vi "Puff_Dose.vi"() -> (5 "Plug in titles":string[](array[string]), 7 "Plug in values":string[](array[string]))   [LabVIEW 2014]
uses:
  Controls/Post_Process.ctl
  <vilib>/Analysis/baseanly.llb/Mean (DBL).vi
  Globals/Meas_global.vi
  Globals/Plug_in_data_global.vi
  <vilib>/Analysis/NI_AALBase.lvlib
panel:
  out "Active Trace length":i32
  out "Background time used (s)":dbl
  out "Delta T":dbl
  out "Min Dose":dbl
  out "Stats Names":string[](array[string])
  out "Stats values":string[](array[string])
  in  "File Extension":string=".xls"
  in  "Save Puff file":bool
  out "Bkgnd value (ppm)":dbl format="%0.2f"
  out "Array":dbl[][](array[numeric])
  out "Puff Number":i32=51
  out "XY Graph":cluster{"Time (s)":dbl[], "Eng Values":dbl[]}[](graph)
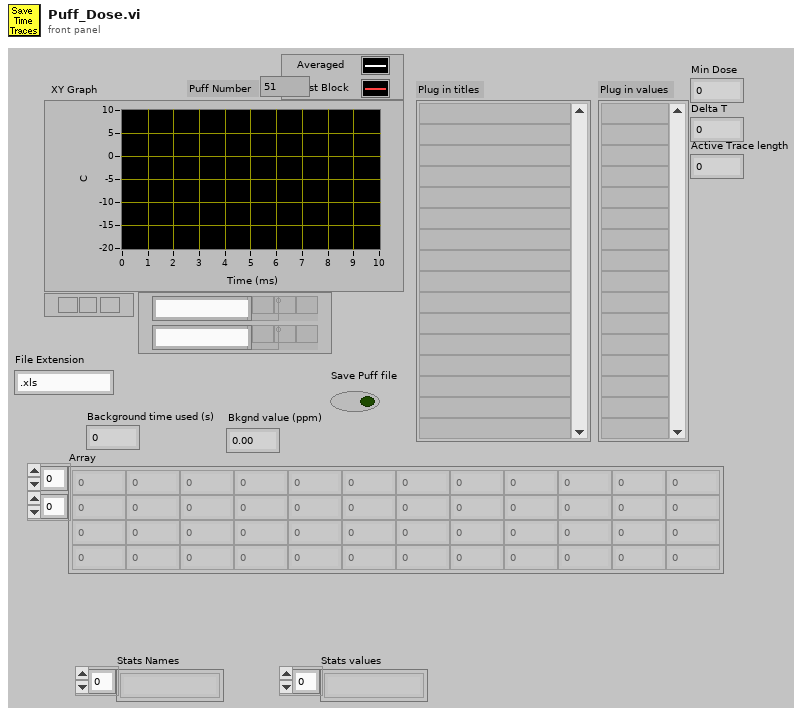
[diagram p1: front panel]
types:
  T1 = typedef "Analysis_info_cluster.ctl" = cluster{"Colour":u32, "Inst type":T2, "Inst name":string, "Symbol":string, "Code name":string, "Extra Info":string, "Inst Array":T3, "Extra Titles":string[], "Extra Values":string[], "U":dbl, "u^2":dbl, "u^3":dbl, "u^4":dbl, "Skew_u":dbl, "Kurt_u":dbl, "Sd Error in Mean":dbl, "% u'/U":dbl, "X":dbl, "Y":dbl, "Z":dbl, "Timescale integral to 25%":dbl, "Sd Error in Variance":dbl, "Calib File":path, "Calib Constants":dbl[], "Output Position":bool, "Full Stats":bool, "Av Sampling Rate":dbl, "Av No of Samples":dbl, "Total Meas Time (s)":dbl, "ADAM Ch Name":string}
  T2 = typedef "Inst_type.ctl" = enum16{"Propeller anemometer", "Raw voltage", "Pressure Transducer", "Pitot-static tube", "Preston tube", "Hot wire", "Cross wire 1", "Cross wire 2", "Generic Linear", "Generic Polynomial", "Generic BackPoly", "Fast FID", "Thermocouple", "Cold wire", "Pulsed Wire", "LDA Vel", "LDA Tran time", "LDA Arr time"}
  T3 = typedef "Instrument_Array.ctl" = enum16{"PWA", "LDA", "Analogue"}
  T4 = typedef "Post_Process.ctl" = enum16{"Take New Data", "Post Process Raw Data File"}
  T5 = enum16{"Save no data", "Save data in new files", "Save data in existing files"}
  T6 = typedef "Time_Trace_Cluster.ctl" = cluster{"Weighting":dbl[], "Time (s)":dbl[], "Voltage":dbl[], "Eng Values":dbl[]}
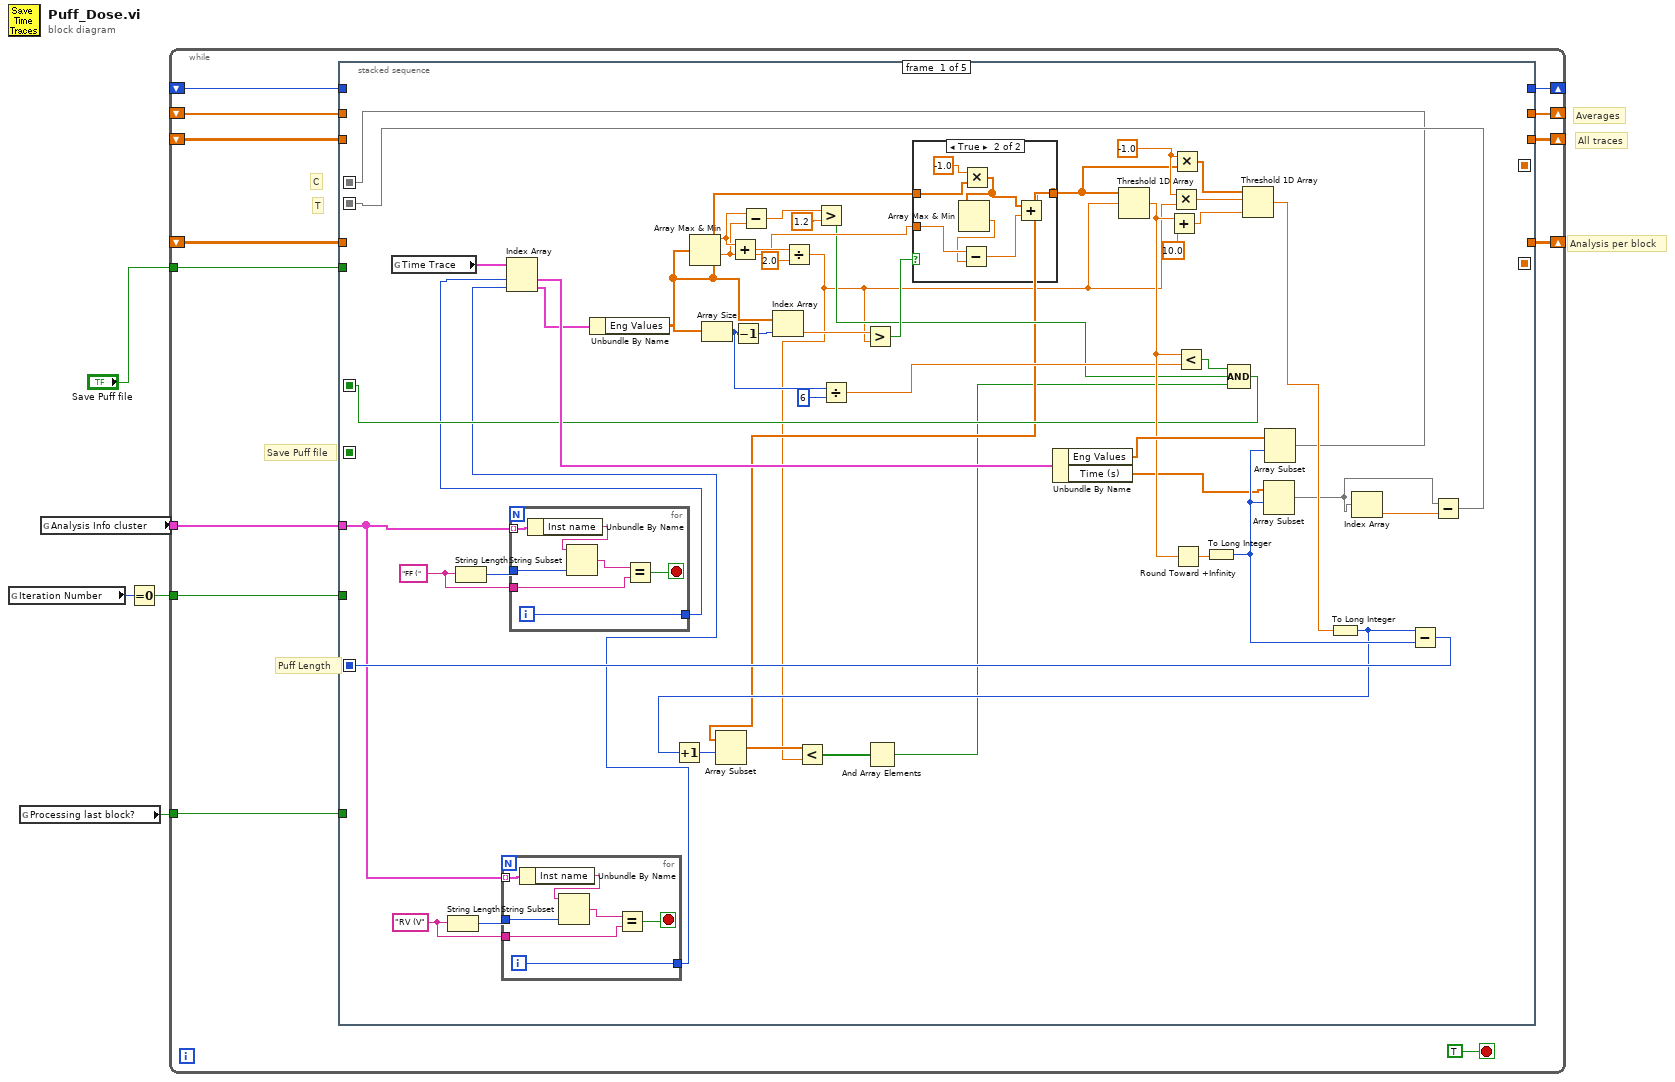
[diagram p0: block diagram]
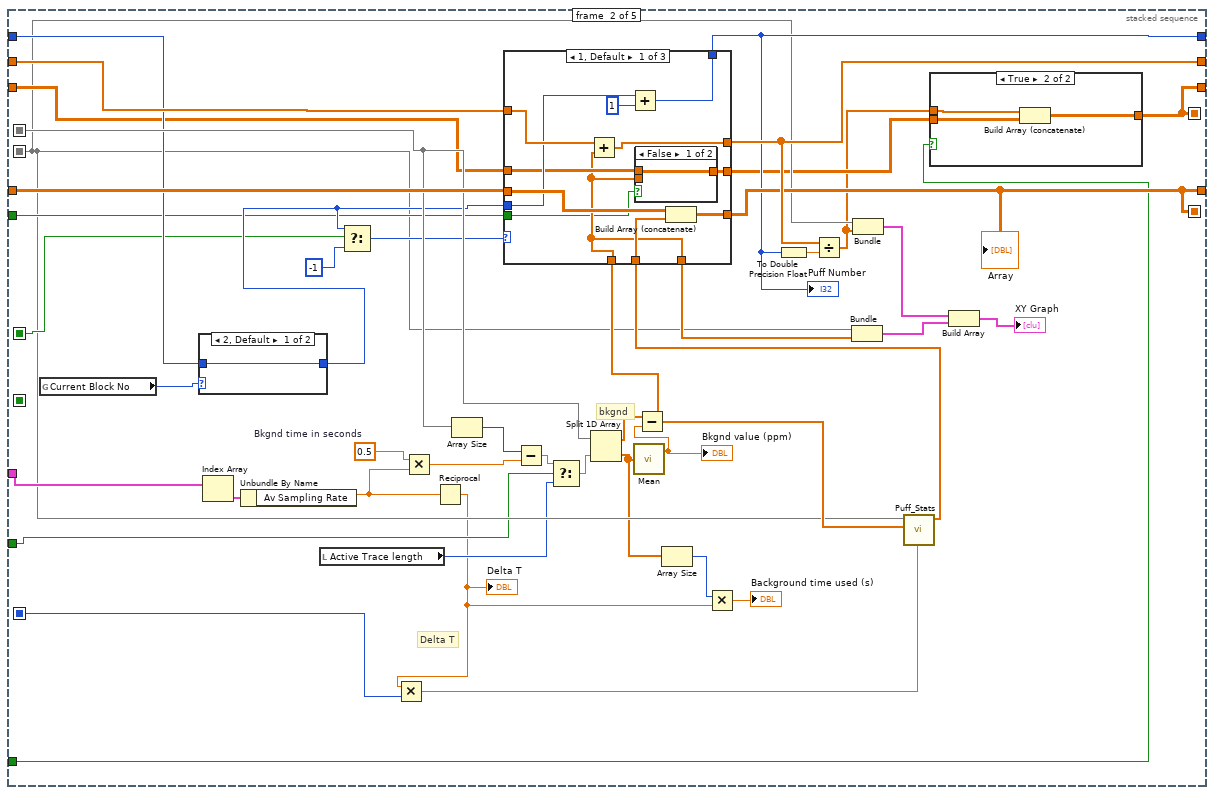
[diagram p3: hidden frame]
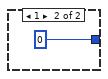
[diagram p5: hidden frame]
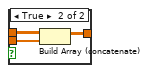
[diagram p6: hidden frame]
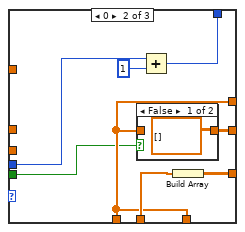
[diagram p7: hidden frame]
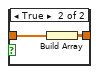
[diagram p8: hidden frame]
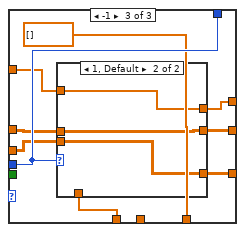
[diagram p9: hidden frame]
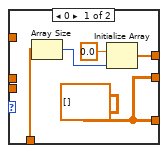
[diagram p10: hidden frame]
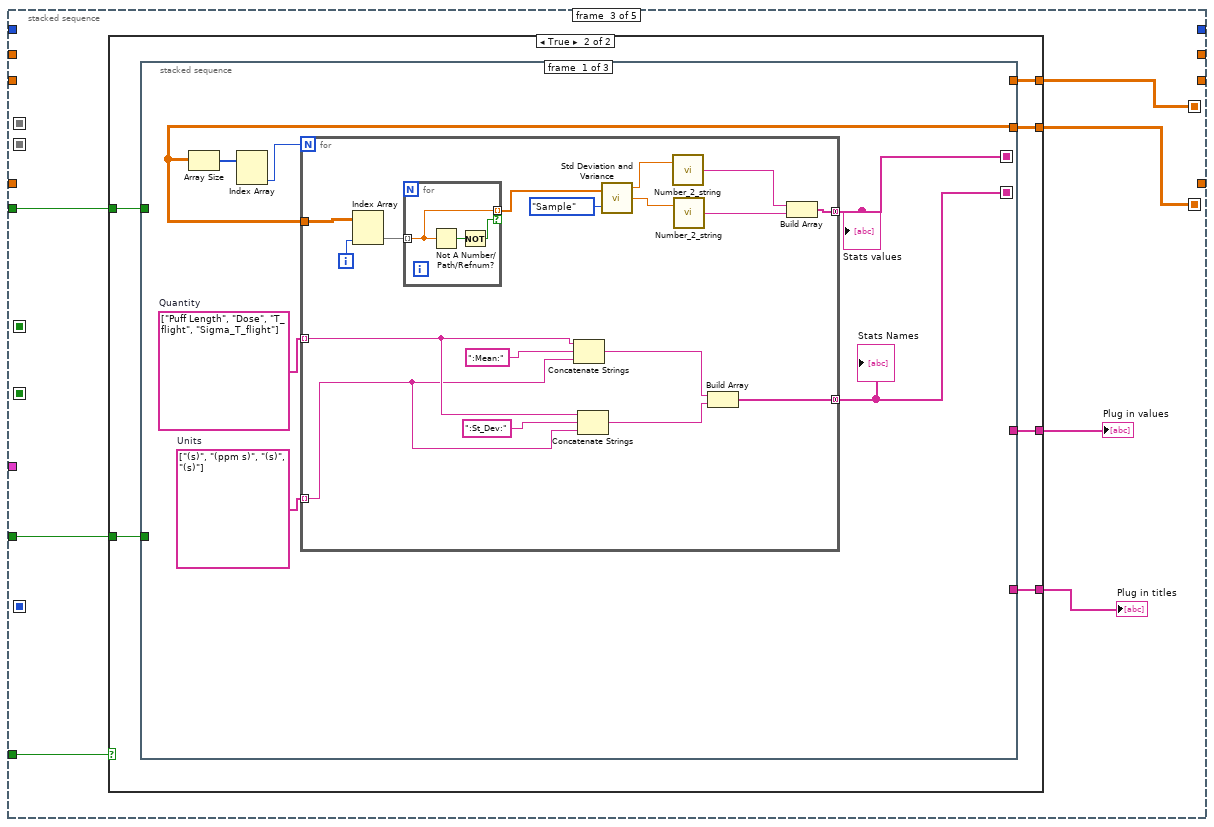
[diagram p11: hidden frame]
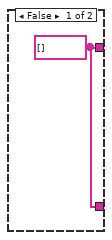
[diagram p12: hidden frame]
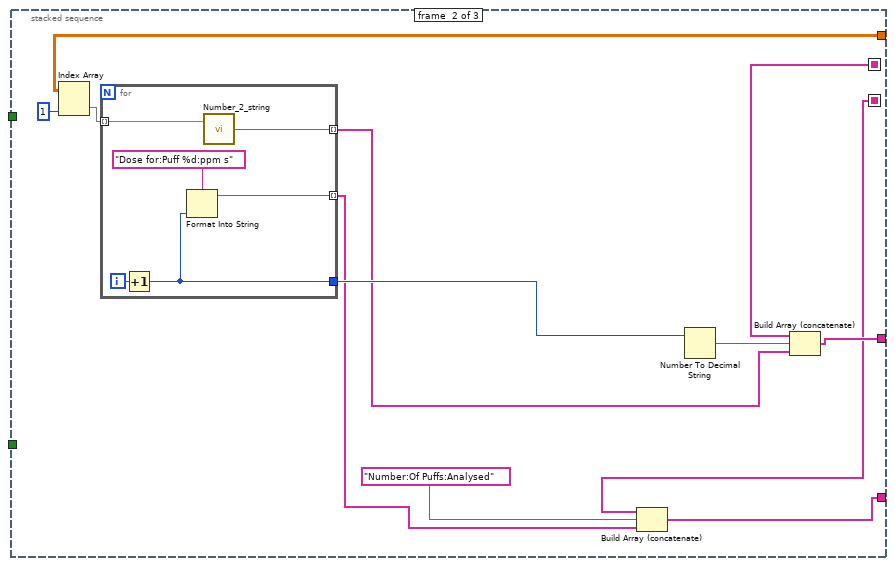
[diagram p13: hidden frame]
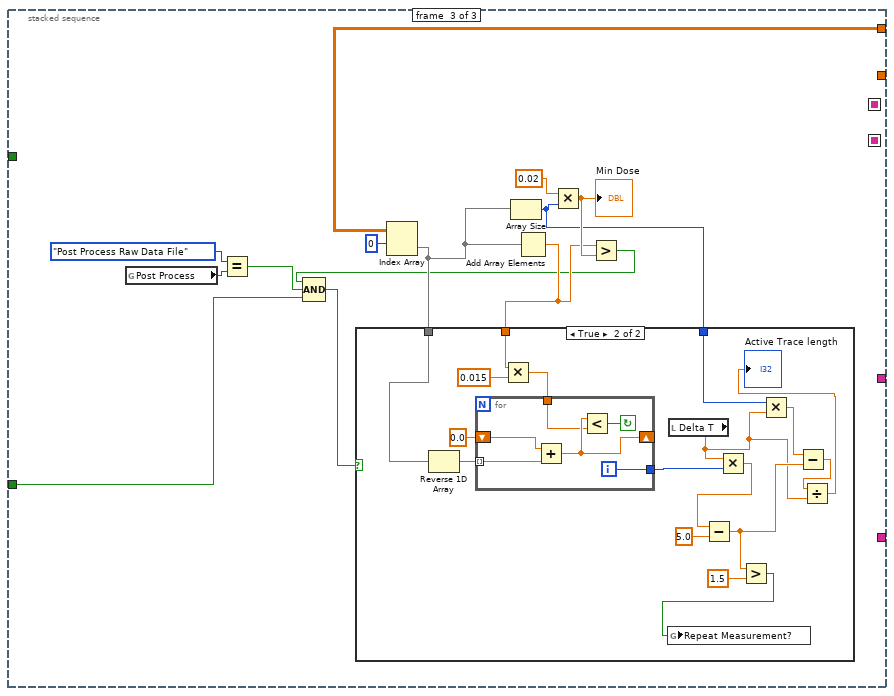
[diagram p14: hidden frame]
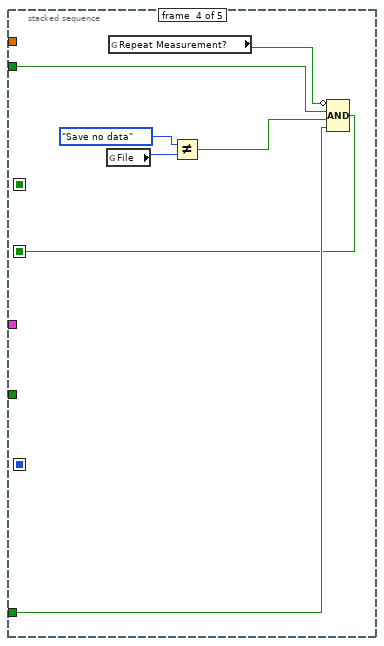
[diagram p16: hidden frame]
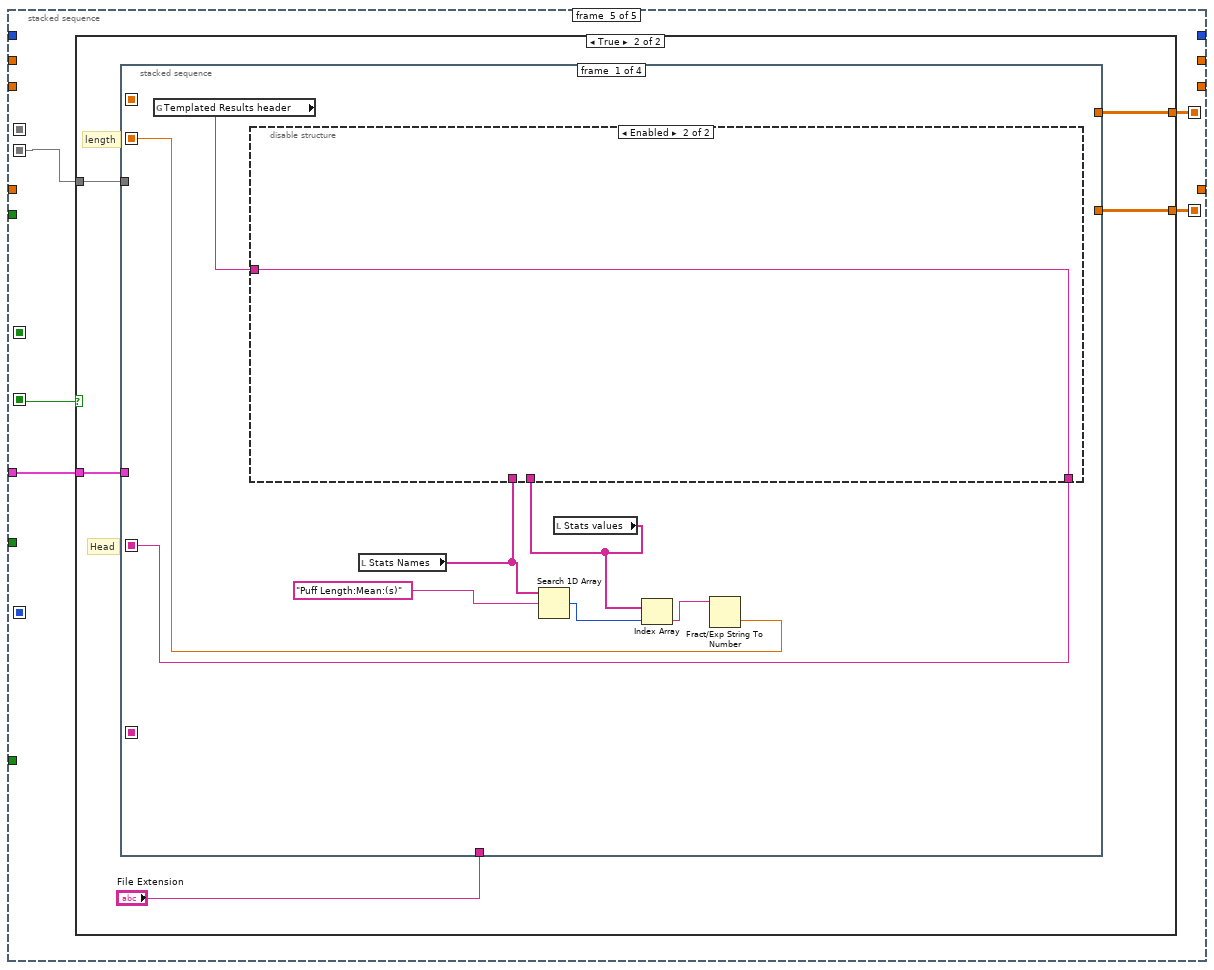
[diagram p17: hidden frame]
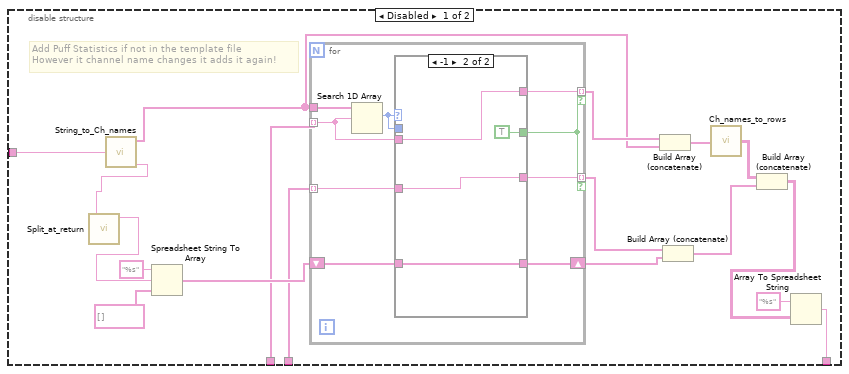
[diagram p19: hidden frame]
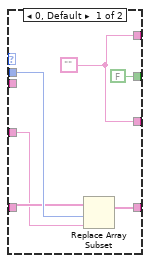
[diagram p20: hidden frame]
diagram:
  # "Averages"
  # "All traces"
  # "Analysis per block"
  n1 = global read "Meas_global.vi" "Iteration Number"() -> (w2:i32)
  n2 = global read "Meas_global.vi" "Processing last block?"() -> (w3:bool)
  n3 = global read "Meas_global.vi" "Analysis Info cluster"() -> (w5:T1[])
  n4 = Equal To 0?(x=w2) -> (x = 0?=w1:bool)
  n5 = while {
    shift-right: [w16] -> _
    shift-left: _ -> [w18]
    shift-right: [w14] -> _
    shift-left: _ -> [w15]
    tunnel: w5 -> [w13]
    shift-right: [w11] -> _
    shift-left: _ -> [w12]
    shift-right: [w10] -> _
    shift-left: _ -> [w9]
    tunnel: "Save Puff file" -> [w8]
    tunnel: w3 -> [w7]
    tunnel: w1 -> [w6]
    stop <- TRUE stop-if-true
    # "Save Puff file"
    # "Puff Length"
    # "T"
    # "C"
    n6 = stacked-sequence {
      seq-local: [_ w121 _ _ _] -> [_ _ w190 _ w289]
      seq-local: [w34 _ _ _ _] -> [_ w120 _ _ _]
      seq-local: [w35 _ _ _ _] -> [_ w103 _ _ w287]
      seq-local: [w33 _ _ _ _] -> [_ w118 _ _ _]
      seq-local: [w38 _ _ _ _] -> [_ w109 _ _ _]
      seq-local: [_ w99 _ _ _] -> [_ _ w184 _ w290]
      seq-local: [_ _ _ w280 _] -> [_ _ _ _ w286]
      tunnel: w18 -> [_ w117 _ _ _]
      tunnel: [_ w132 _ _ _] -> w16
      tunnel: w15 -> [_ w122 _ _ _]
      tunnel: [_ w121 _ _ _] -> w14
      tunnel: w13 -> [w21 w119 _ _ w288]
      tunnel: w12 -> [_ w115 _ _ _]
      tunnel: [_ w114 _ _ _] -> w11
      tunnel: [_ w99 _ _ _] -> w10
      tunnel: w9 -> [_ w105 _ _ _]
      tunnel: w8 -> [_ w104 w187 w283 _]
      tunnel: w7 -> [_ w102 w186 w281 _]
      tunnel: w6 -> [_ w96 w185 _ _]
      frame #0 {
        w23 = "RV (V"
        w58 = -1.0
        w65 = "FF ("
        n7 = global read "Meas_global.vi" "Time Trace"() -> (w67:T6[])
        n8 = String Length(string=w23) -> (length=w22:i32)
        n9 = String Length(string=w65) -> (length=w66:i32)
        n10 = for {
          tunnel: w21 -> [w74] mode=indexing
          tunnel: w22 -> [w73]
          tunnel: w23 -> [w70]
          tunnel: [w68] -> w20
          i -> [w68]
          stop <- w69 stop-if-true
          n11 = Unbundle By Name(w74) -> ("Inst name"=w72:string)
          n12 = String Subset(string=w72, length (rest)=w73) -> (substring=w71:string)  [unwired: 1 in]
          n13 = Equal?(x=w71, y=w70) -> (x = y?=w69:bool)
        }
        n14 = for {
          tunnel: w21 -> [w89] mode=indexing
          tunnel: w66 -> [w88]
          tunnel: w65 -> [w85]
          tunnel: [w83] -> w19
          i -> [w83]
          stop <- w84 stop-if-true
          n15 = Unbundle By Name(w89) -> ("Inst name"=w87:string)
          n16 = String Subset(string=w87, length (rest)=w88) -> (substring=w86:string)  [unwired: 1 in]
          n17 = Equal?(x=w86, y=w85) -> (x = y?=w84:bool)
        }
        n18 = Index Array(array=w67, index #1=w19, index #2=w20) -> (element #1=w64:T6, element #2=w63:T6)
        n19 = Unbundle By Name(w63) -> ("Eng Values"=w30:dbl[])
        n20 = Array Max & Min(array=w30) -> (max value=w48:dbl, min value=w47:dbl)  [unwired: 2 out]
        n21 = Array Size(array=w30) -> (size(s)=w43:i32)
        n22 = Add(x=w48, y=w47) -> (x+y=w62:dbl)
        n23 = Decrement(x=w43) -> (x-1=w52:i32)
        n24 = Subtract(x=w48, y=w47) -> (x-y=w46:dbl)
        n25 = Index Array(array=w30, index=w52) -> (element=w51:dbl)
        n26 = Divide(x=w62, y=2.0) -> (x/y=w26:dbl)
        n27 = Greater?(x=w46, y=1.2) -> (0:w39:bool)
        n28 = Divide(x=w43, y=6) -> (x/y=w41:dbl)
        n29 = Greater?(x=w51, y=w26) -> (0:w50:bool)
        n30 = case shown="True" w50 {
          tunnel: w30 -> [w75 w81]
          tunnel: [w75 w76] -> w28
          tunnel: w47 -> [_ w80]
          frame False {
          }
          frame True {
            n31 = Multiply(x=-1.0, y=w81) -> (x*y=w77:dbl[])
            n32 = Array Max & Min(array=w77) -> (min value=w79:dbl)  [unwired: 3 out]
            n33 = Subtract(x=w80, y=w79) -> (x-y=w78:dbl)
            n34 = Add(x=w77, y=w78) -> (x+y=w76:dbl[])
          }
        }
        n35 = Unbundle By Name(w64) -> ("Eng Values"=w55:dbl[], "Time (s)"=w31:dbl[])
        n36 = Threshold 1D Array(2:w26, 3:w28) -> (0:w44:dbl)  [unwired: 1 in]
        n37 = Add(x=w44, y=10.0) -> (x+y=w60:dbl)
        n38 = Multiply(x=w58, y=w26) -> (x*y=w57:dbl)
        n39 = Multiply(x=w58, y=w28) -> (x*y=w49:dbl[])
        n40 = Round Toward +Infinity(x=w44) -> (ceil(x): smallest int >= x=w56:dbl)
        n41 = Less?(x=w44, y=w41) -> (x < y?=w40:bool)
        n42 = To Long Integer(number=w56) -> (32bit integer=w53:i32)
        n43 = Threshold 1D Array(1:w60, 2:w57, 3:w49) -> (0:w54:dbl)
        n44 = Array Subset(array=w31, index=w53) -> (w36:dbl[])  [unwired: 1 in]
        n45 = Array Subset(array=w55, index=w53) -> (w34:dbl[])  [unwired: 1 in]
        n46 = To Long Integer(number=w54) -> (32bit integer=w32:i32)
        n47 = Increment(x=w32) -> (x+1=w29:i32)
        n48 = Array Subset(array=w28, index=w29) -> (w27:dbl[])  [unwired: 1 in]
        n49 = Less?(x=w27, y=w26) -> (x < y?=w25:bool[])
        n50 = And Array Elements(Boolean array=w25) -> (logical AND=w24:bool)
        n51 = Compound Arithmetic op=AND(w40, w39, w24) -> (w38:bool)
        n52 = Index Array(array=w36) -> (element=w37:dbl)  [unwired: 1 in]
        n53 = Subtract(x=w32, y=w53) -> (x-y=w33:i32)
        n54 = Subtract(x=w36, y=w37) -> (x-y=w35:dbl[])
      }
      frame #1 {
        w90 = 0.5  # Bkgnd time in seconds
        # "bkgnd"
        # "Delta T"
        n55 = global read "Meas_global.vi" "Current Block No"() -> (w116:i32)
        n56 = case shown="2, Default" w116 {
          tunnel: [w138 0] -> w113
          tunnel: w115 -> [w138 _]
          frame 2, Default {
          }
          frame 1 {
          }
        }
        n57 = Index Array(array=w119) -> (element=w128:T1)  [unwired: 1 in]
        n58 = Unbundle By Name(w128) -> ("Av Sampling Rate"=w123:dbl)
        n59 = local read "Active Trace length"() -> (w95:i32)
        n60 = Select(t=w113, s=w109, f=-1) -> (s? t:f=w111:i32)
        n61 = Multiply(x=w90, y=w123) -> (x*y=w126:dbl)
        n62 = Reciprocal(x=w123) -> (1/x=w91:dbl)
        "Delta T" <- w91
        n63 = Multiply(x=w91, y=w118) -> (x*y=w108:dbl)
        n64 = Array Size(array=w120) -> (size(s)=w127:i32)
        n65 = Subtract(x=w127, y=w126) -> (x-y=w98:dbl)
        n66 = Select(t=w98, s=w96, f=w95) -> (s? t:f=w97:dbl)
        n67 = Split 1D Array(array=w120, index=w97) -> (first subarray=w124:dbl[], second subarray=w94:dbl[])
        n68 = call-poly <vilib>:"Mean.vi"("X"=w94) -> ("mean"=w125:dbl)  [unwired: 1 out]
        "Bkgnd value (ppm)" <- w125
        n69 = Subtract(x=w124, y=w125) -> (x-y=w107:dbl[])
        n70 = Array Size(array=w94) -> (size(s)=w93:i32)
        n71 = Multiply(x=w93, y=w91) -> (x*y=→"Background time used (s)":dbl)
        n72 = call "Puff_Stats.vi"("Puff release time (s)"=w108, "Concentrations"=w107, "Time (s)"=w103) -> ("Stats"=w110:dbl[])  [unwired: 8 in]
        n73 = case shown="1, Default" w111 {
          tunnel: [w150 w158 w174] -> w132
          tunnel: w117 -> [w151 _ w173]
          tunnel: w110 -> [w149 w163 _]
          tunnel: [w148 w162 w169] -> w121
          tunnel: w122 -> [w147 _ w172]
          tunnel: w113 -> [w144 w161 w175]
          tunnel: [w145 w159 w175] -> w114
          tunnel: w107 -> [w142 w158 w171]
          tunnel: [w142 w158 dbl[] []] -> w106
          tunnel: [w141 w157 w168] -> w101
          tunnel: w105 -> [w143 _ w167]
          tunnel: w104 -> [w140 w156 _]
          frame 1, Default {
            n74 = Add(x=w151, y=w142) -> (x+y=w150:dbl[])
            n75 = Add(x=w144, y=1) -> (x+y=w145:i32)
            n76 = case shown="False" w140 {
              tunnel: w143 -> [w152 w155]
              tunnel: w142 -> [_ w154]
              tunnel: [w152 w153] -> w141
              frame False {
              }
              frame True {
                n77 = Build Array (concatenate)(w155, w154) -> (w153:dbl[][])
              }
            }
            n78 = Build Array (concatenate)(w147, w149) -> (w148:dbl[][])
          }
          frame 0 {
            n79 = case shown="False" w156 {
              tunnel: w158 -> [_ w166]
              tunnel: [dbl[][] [] w165] -> w157
              frame False {
              }
              frame True {
                n80 = Build Array(w166) -> (w165:dbl[][])
              }
            }
            n81 = Add(x=w161, y=1) -> (x+y=w159:i32)
            n82 = Build Array(w163) -> (w162:dbl[][])
          }
          frame -1 {
            n83 = case shown="1, Default" w175 {
              tunnel: w171 -> [w180 _]
              tunnel: [w177 w183] -> w174
              tunnel: [w176 w182] -> w169
              tunnel: w173 -> [_ w183]
              tunnel: w172 -> [_ w182]
              tunnel: [w176 w181] -> w168
              tunnel: w167 -> [_ w181]
              frame 0 {
                w176 = dbl[][] []
                n84 = Array Size(array=w180) -> (size(s)=w179:i32)
                n85 = Initialize Array(0.0 ("element"), w179) -> (w177:dbl[])
              }
              frame 1, Default {
              }
            }
          }
        }
        "Puff Number" <- w114
        "Array" <- w121
        n86 = To Double Precision Float(number=w114) -> (double precision float=w133:dbl)
        n87 = Divide(x=w132, y=w133) -> (x/y=w100:dbl[])
        n88 = Bundle(w103, w106) -> (w131:cluster{dbl[], dbl[]})  [unwired: 1 in]
        n89 = Bundle(w103, w100) -> (w130:cluster{dbl[], dbl[]})  [unwired: 1 in]
        n90 = case shown="True" w102 {
          tunnel: w101 -> [w134 w137]
          tunnel: w100 -> [_ w136]
          tunnel: [w134 w135] -> w99
          frame False {
          }
          frame True {
            n91 = Build Array (concatenate)(w136, w137) -> (w135:dbl[][])
          }
        }
        n92 = Build Array(w130, w131) -> (→"XY Graph":cluster{dbl[], dbl[]}[])
      }
      frame #2 {
        n93 = case shown="True" w186 {
          tunnel: w190 -> [_ w197]
          tunnel: [w191 w196] -> w189
          tunnel: [w191 w195] -> w188
          tunnel: w187 -> [_ w194]
          tunnel: w185 -> [_ w193]
          tunnel: w184 -> [_ w192]
          frame False {
            w191 = string[] []
          }
          frame True {
            n94 = stacked-sequence {
              seq-local: [w199 _ _] -> [_ w231 _]
              seq-local: [w198 _ _] -> [_ w230 _]
              tunnel: w197 -> [w202 w234 _]
              tunnel: [_ w236 _] -> w196
              tunnel: [_ w235 _] -> w195
              tunnel: w194 -> [_ _ _]
              tunnel: w193 -> [_ _ w252]
              tunnel: w192 -> [_ _ w251]
              frame #0 {
                w200 = string[] ["(s)", "(ppm s)", "(s)", "(s)"]  # Units
                w201 = string[] ["Puff Length", "Dose", "T_flight", "Sigma_T_flight"]  # Quantity
                n95 = Array Size(array=w202) -> (size(s)=w204:i32[])
                n96 = Index Array(array=w204) -> (element #2=w203:i32)  [unwired: 2 in, 1 out]
                n97 = for {
                  N: w203 -> [_]
                  tunnel: w202 -> [w221]
                  tunnel: w201 -> [w212] mode=indexing
                  tunnel: w200 -> [w211] mode=indexing
                  tunnel: [w208] -> w199 mode=concatenating
                  tunnel: [w207] -> w198 mode=concatenating
                  i -> [w220]
                  n98 = Index Array(array=w221, index (col)=w220) -> (element=w206:dbl[])  [unwired: 1 in]
                  n99 = for {
                    tunnel: w206 -> [w224] mode=indexing
                    tunnel: [w224] -> w205 mode=indexing if=w222
                    n100 = Not A Number/Path/Refnum?(number/path/refnum=w224) -> (NaN/Path/Refnum?=w223:bool)
                    n101 = Not(x=w223) -> (.not. x?=w222:bool)
                  }
                  n102 = Concatenate Strings(w212, ":Mean:" ("string"), w211) -> (w209:string)
                  n103 = Concatenate Strings(w212, ":St_Dev:" ("string"), w211) -> (w210:string)
                  n104 = call <vilib>:"Std Deviation and Variance.vi"("X"=w205, "Weighting (Sample)"=enum16{"Sample", "Population"}."Sample") -> ("mean"=w217:dbl, "standard deviation"=w218:dbl)  [unwired: 1 out]
                  n105 = call "Number_2_string.vi"("number"=w217) -> ("String"=w216:string)  [unwired: 1 in]
                  n106 = call "Number_2_string.vi"("number"=w218) -> ("String"=w215:string)  [unwired: 1 in]
                  n107 = Build Array(w209, w210) -> (w207:string[])
                  n108 = Build Array(w216, w215) -> (w208:string[])
                }
                "Stats values" <- w199
                "Stats Names" <- w198
              }
              frame #1 {
                n109 = Index Array(array=w234, index (col)=1 ("disabled index (col)")) -> (element=w232:dbl[])  [unwired: 1 in]
                n110 = for {
                  tunnel: w232 -> [w242] mode=indexing
                  tunnel: [w239] -> w227 mode=indexing
                  tunnel: [w238] -> w226 mode=indexing
                  tunnel: [w237] -> w229
                  i -> [w241]
                  n111 = Increment(x=w241) -> (x+1=w237:i32)
                  n112 = Format Into String(format string="Dose for:Puff %d:ppm s", w237) -> (resulting string=w238:string)  [unwired: 2 in, 1 out]
                  n113 = call "Number_2_string.vi"("number"=w242) -> ("String"=w239:string)  [unwired: 1 in]
                }
                n114 = Build Array (concatenate)(w230, "Number:Of Puffs:Analysed" ("format string"), w226) -> (w235:string[])
                n115 = Number To Decimal String(number=w229) -> (decimal integer string=w228:string)  [unwired: 1 in]
                n116 = Build Array (concatenate)(w231, w228, w227) -> (w236:string[])
              }
              frame #2 {
                n117 = global read "Meas_global.vi" "Post Process"() -> (w255:T4)
                n118 = Equal?(x=Post_Process."Post Process Raw Data File" ("Post Process"), y=w255) -> (x = y?=w253:bool)
                n119 = Index Array(array=w251, index (row)=0) -> (element=w249:dbl[])  [unwired: 1 in]
                n120 = Array Size(array=w249) -> (size(s)=w243:i32)
                n121 = Add Array Elements(numeric array=w249) -> (sum=w246:dbl)
                n122 = Multiply(x=0.02, y=w243) -> (x*y=w247:dbl)
                "Min Dose" <- w247
                n123 = Greater?(x=w246, y=w247) -> (0:w245:bool)
                n124 = Compound Arithmetic op=AND(w245, w253, w252) -> (w244:bool)
                n125 = case shown="True" w244 {
                  tunnel: w249 -> [_ w270]
                  tunnel: w246 -> [_ w269]
                  tunnel: w243 -> [_ w261]
                  frame False {
                  }
                  frame True {
                    n126 = Reverse 1D Array(array=w270) -> (reversed array=w272:dbl[])
                    n127 = Multiply(x=w269, y=0.015) -> (x*y=w267:dbl)
                    n128 = for {
                      shift-right: [w276] -> _
                      shift-left: 0.0 -> [w277]
                      tunnel: w272 -> [w278] mode=indexing
                      tunnel: w267 -> [w275]
                      tunnel: [w273] -> w262
                      i -> [w273]
                      stop <- w274 continue-if-true
                      n129 = Add(x=w277, y=w278) -> (x+y=w276:dbl)
                      n130 = Less?(x=w276, y=w275) -> (x < y?=w274:bool)
                    }
                    n131 = local read "Delta T"() -> (w257:dbl)
                    n132 = Multiply(x=w257, y=w262) -> (x*y=w266:dbl)
                    n133 = Subtract(x=w266, y=5.0) -> (x-y=w259:dbl)
                    n134 = Greater?(x=w259, y=1.5) -> (0:w263:bool)
                    n135 = global write "Meas_global.vi" "Repeat Measurement?"(w263) -> ()
                    n136 = Multiply(x=w261, y=w257) -> (x*y=w260:dbl)
                    n137 = Subtract(x=w260, y=w259) -> (x-y=w258:dbl)
                    n138 = Divide(x=w258, y=w257) -> (x/y=→"Active Trace length":dbl)
                  }
                }
              }
            }
          }
        }
        "Plug in titles" <- w188
        "Plug in values" <- w189
      }
      frame #3 {
        n139 = global read "Meas_global.vi" "File"() -> (w285:T5)
        n140 = global read "Meas_global.vi" "Repeat Measurement?"() -> (w279:bool)
        n141 = Not Equal?(x=T5."Save no data" ("File"), y=w285) -> (x != y?=w282:bool)
        n142 = Compound Arithmetic op=AND(invert w279, w283, w282, w281) -> (w280:bool)
      }
      frame #4 {
        n143 = case shown="True" w286 {
          tunnel: w290 -> [_ w295]
          tunnel: w289 -> [_ w294]
          tunnel: w288 -> [_ w293]
          tunnel: w287 -> [_ w292]
          frame False {
          }
          frame True {
            # "Head"
            # "length"
            n144 = stacked-sequence {
              seq-local: [_ w366 _ _] -> [_ _ w401 _]
              seq-local: [w298 _ _ _] -> [_ _ w403 w453]
              seq-local: [w300 _ _ _] -> [_ w354 _ _]
              seq-local: [_ w342 _ _] -> [_ _ _ w418]
              tunnel: w295 -> [_ w346 _ _]
              tunnel: w294 -> [_ w352 _ _]
              tunnel: w293 -> [_ _ _ _]
              tunnel: w292 -> [_ w355 _ w419]
              tunnel: "File Extension" -> [_ _ w399 w421]
              frame #0 {
                n145 = global read "Plug_in_data_global.vi" "Templated Results header"() -> (w299:string)
                n146 = local read "Stats Names"() -> (w297:string[])
                n147 = Search 1D Array(1D array=w297, element="Puff Length:Mean:(s)") -> (index of element=w302:i32)  [unwired: 1 in]
                n148 = local read "Stats values"() -> (w296:string[])
                n149 = disable-structure shown="Enabled" {
                  disable-tunnel: w297 -> [w307 _]
                  disable-tunnel: w296 -> [w306 _]
                  disable-tunnel: w299 -> [w305 w341]
                  disable-tunnel: [w304 w341] -> w298
                  frame Disabled {
                    # "Add Puff Statistics if not in the template file\nHowever it channel name changes it adds it again!"
                    n150 = call "String_to_Ch_names.vi"("Spreadsheet string"=w305) -> ("Ch names"=w310:string[], "String After names"=w320:string)  [unwired: 2 out]
                    n151 = call "Split_at_return.vi"("String"=w320) -> ("before substring"=w321:string)  [unwired: 1 in, 3 out]
                    n152 = Spreadsheet String To Array(format string="%s", spreadsheet string=w321, array type (2D Dbl)=string[] [] ("Channel Values")) -> (array=w317:string[])  [unwired: 1 out]
                    n153 = for {
                      tunnel: w310 -> [w330]
                      tunnel: w307 -> [w329] mode=indexing
                      tunnel: [w328] -> w316 mode=indexing if=w323
                      tunnel: [w327] -> w315 mode=indexing if=w323
                      tunnel: w306 -> [w326] mode=indexing
                      shift-right: [w325] -> w314
                      shift-left: w317 -> [w324]
                      n154 = Search 1D Array(1D array=w330, element=w329) -> (index of element=w322:i32)  [unwired: 1 in]
                      n155 = case shown="-1" w322 {
                        tunnel: w329 -> [_ w340]
                        tunnel: [w335 w340] -> w328
                        tunnel: [w335 w339] -> w327
                        tunnel: w326 -> [w331 w339]
                        tunnel: [w332 w338] -> w325
                        tunnel: w324 -> [w333 w338]
                        tunnel: [FALSE TRUE] -> w323
                        tunnel: w322 -> [w334 _]
                        frame 0, Default {
                          w335 = ""
                          n156 = Replace Array Subset(array=w333, new element=w331, index=w334) -> (w332:string[])
                        }
                        frame -1 {
                        }
                      }
                    }
                    n157 = Build Array (concatenate)(w316, w310) -> (w312:string[])
                    n158 = Build Array (concatenate)(w315, w314) -> (w313:string[])
                    n159 = call "Ch_names_to_rows.vi"("Channel Names"=w312) -> ("3 Row names"=w311:string[][])
                    n160 = Build Array (concatenate)(w311, w313) -> (w308:string[][])
                    n161 = Array To Spreadsheet String(array=w308, 3:"%s" ("format string")) -> (spreadsheet string=w304:string)  [unwired: 1 in]
                  }
                  frame Enabled {
                  }
                }
                n162 = Index Array(array=w296, index=w302) -> (element=w301:string)
                n163 = Fract/Exp String To Number(string=w301) -> (number=w300:dbl)  [unwired: 3 in, 1 out]
              }
              frame #1 {
                w359 = ""
                n164 = Array Size(array=w346) -> (size(s)=w370:i32[])
                n165 = Index Array(array=w370) -> (element #1=w343:i32, element #2=w344:i32)  [unwired: 2 in]
                n166 = for {
                  N: w344 -> [_]
                  tunnel: w346 -> [w376]
                  tunnel: w343 -> [w374]
                  tunnel: [w373] -> w345 mode=indexing
                  i -> [w375]
                  n167 = for {
                    N: w374 -> [_]
                    tunnel: w376 -> [w385]
                    tunnel: w375 -> [w384]
                    tunnel: [w377] -> w373 mode=indexing
                    i -> [w383]
                    n168 = Index Array(array=w385, index (row)=w383, index (col)=w384) -> (element=w378:dbl)
                    n169 = Equal To 0?(x=w383) -> (x = 0?=w382:bool)
                    n170 = Select(t=i16 3, s=w382, f=i16 1 ("precision (6)")) -> (s? t:f=w379:i16)
                    n171 = Number To Fractional String(number=w378, precision (6)=w379) -> (F-format string=w377:string)  [unwired: 2 in]
                  }
                }
                n172 = for {
                  N: w344 -> [_]
                  tunnel: w355 -> [w390] mode=indexing
                  tunnel: [w389] -> w360 mode=indexing
                  n173 = call "Number_2_string.vi"("number"=w390) -> ("String"=w389:string)  [unwired: 1 in]
                }
                n174 = for {
                  N: w343 -> [_]
                  tunnel: [w393] -> w350 mode=indexing
                  tunnel: [""] -> w357 mode=indexing
                  i -> [w391]
                  n175 = Format Into String(format string="Puff_%d", w391) -> (resulting string=w393:string)  [unwired: 2 in, 1 out]
                }
                n176 = Index Array(array=w346, index (row)=0) -> (element=w342:dbl[])  [unwired: 1 in]
                n177 = Build Array (concatenate)(w359, "Puff_Length (s)", "Puff_Dose (ppm s)", "T_flight (s)", "Sigma_T_flight (s)", w359, "Time (s)", w360) -> (w369:string[])
                n178 = call "Puff_Stats.vi"("Puff release time (s)"=w354, "Concentrations"=w342, "Time (s)"=w355) -> ("Stats"=w353:dbl[])  [unwired: 8 in]
                n179 = Replace Array Subset(array=w350, new element="Averaged Puff", index=0) -> (w349:string[])
                n180 = Build Array (concatenate)(w353, w352) -> (w351:dbl[][])
                n181 = Transpose 2D Array(2D array=w351) -> (transposed array=w372:dbl[][])
                n182 = for {
                  tunnel: w372 -> [w396] mode=indexing
                  tunnel: [w395] -> w371 mode=indexing
                  n183 = for {
                    tunnel: w396 -> [w398] mode=indexing
                    tunnel: [w397] -> w395 mode=indexing
                    n184 = call "Number_2_string.vi"("number"=w398) -> ("String"=w397:string)  [unwired: 1 in]
                  }
                }
                n185 = Build Array (concatenate)(w349, w371, w357, w349, w345) -> (w368:string[][])
                n186 = for {
                  tunnel: w369 -> [w386] mode=indexing
                  tunnel: w368 -> [w388] mode=indexing
                  tunnel: [w387] -> w367 mode=indexing
                  n187 = Build Array (concatenate)(w386, w388) -> (w387:string[])
                }
                n188 = Array To Spreadsheet String(array=w367, 3:"%s" ("format string")) -> (spreadsheet string=w366:string)  [unwired: 1 in]
              }
              frame #2 {
                w402 = "\r\n"
                n189 = global read "Meas_global.vi" "Results file"() -> (w416:path)
                n190 = Strip Path(path=w416) -> (stripped path=w415:path)  [unwired: 1 out]
                n191 = global read "Meas_global.vi" "Raw data file"() -> (w412:path)
                n192 = Strip Path(path=w412) -> (name=w413:string)  [unwired: 1 out]
                n193 = Build Path(base path=w415, name or relative path="Puff_Analysis") -> (appended path=w411:path)
                n194 = call "Add_filename_suffix.vi"("Filename"=w413) -> ("Base name"=w410:string)  [unwired: 1 in, 3 out]
                n195 = Concatenate Strings(w410, w399) -> (w409:string)
                n196 = Build Path(base path=w411, name or relative path=w409) -> (appended path=w408:path)
                n197 = Concatenate Strings(w403, w402, w402, w401) -> (w400:string)
                n198 = call "Find_Unique_Filename.vi"("Path In"=w408, "Max Length (31)"=51) -> ("Unique Path Out"=w406:path)  [unwired: 1 in]
                n199 = call "Create_directory_path.vi"("Path name"=w406) -> ("Path name Out"=w405:path)  [unwired: 1 in, 1 out]
                n200 = call "Write_File_Simple.vi"("append to file? (new file:F)"=FALSE, "character string"=w400, "file path"=w405) -> ()  [unwired: 2 out]
              }
              frame #3 {
                w437 = "\r\n"
                n201 = global read "Meas_global.vi" "Results file"() -> (w435:path)
                n202 = Array Size(array=w418) -> (size(s)=w420:i32)
                n203 = Divide(x=w420, y=100) -> (x/y=w456:dbl)
                n204 = Array Subset(array=w419, length=w420) -> (w417:dbl[])  [unwired: 1 in]
                n205 = Strip Path(path=w435) -> (stripped path=w434:path)  [unwired: 1 out]
                n206 = To Long Integer(number=w456) -> (32bit integer=w455:i32)
                n207 = global read "Meas_global.vi" "Raw data file"() -> (w431:path)
                n208 = call "Downsampler.vi"("Input Array"=w418, "Averaging samples"=w455) -> ("Downsampled Array"=w443:dbl[])  [unwired: 1 out]
                n209 = call "Downsampler.vi"("Input Array"=w417, "Averaging samples"=w455) -> ("Downsampled Array"=w444:dbl[])  [unwired: 1 out]
                n210 = Strip Path(path=w431) -> (name=w432:string)  [unwired: 1 out]
                n211 = Initialize Array("", 10) -> (w450:string[])
                n212 = Build Path(base path=w434, name or relative path="Av_Puff_Plots") -> (appended path=w430:path)
                n213 = Build Array(w444, w443) -> (w442:dbl[][])
                n214 = call "Add_filename_suffix.vi"("Filename"=w432) -> ("Base name"=w429:string)  [unwired: 1 in, 3 out]
                n215 = call "Asterisk_header.vi"("Channel names"=w450) -> ("Header string"=w449:string)
                n216 = Transpose 2D Array(2D array=w442) -> (transposed array=w440:dbl[][])
                n217 = Concatenate Strings(w429, w421) -> (w428:string)
                n218 = Concatenate Strings("Time (s)", "\t", "Av_Puff (ppm)") -> (w445:string)
                n219 = Number To Fractional String(number=w440, precision (6)=i16 3) -> (F-format string=w438:string[][])  [unwired: 2 in]
                n220 = Build Path(base path=w430, name or relative path=w428) -> (appended path=w427:path)
                n221 = Array To Spreadsheet String(array=w438, 3:"%s" ("format string")) -> (spreadsheet string=w436:string)  [unwired: 1 in]
                n222 = Concatenate Strings(w437, "*****This is a many rows per single point file*****", w437, w453, w437, w449, w445, w437, w437, w437, w436) -> (w422:string)
                n223 = call "Find_Unique_Filename.vi"("Path In"=w427, "Max Length (31)"=51) -> ("Unique Path Out"=w425:path)  [unwired: 1 in]
                n224 = call "Create_directory_path.vi"("Path name"=w425) -> ("Path name Out"=w424:path)  [unwired: 1 in, 1 out]
                n225 = call "Write_File_Simple.vi"("append to file? (new file:F)"=FALSE, "character string"=w422, "file path"=w424) -> ()  [unwired: 2 out]
              }
            }
          }
        }
      }
    }
  }
